vi "add channel to active arrayv2.vi"(0 "line array in":u32[](array[numeric]), 1 "line to add":u32) -> (2 "line array out":u32[](array[numeric]), 3 "addition":bool, 4 "index":i32)   [LabVIEW 2015]
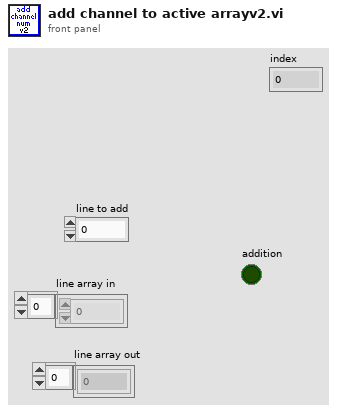
[diagram p1: front panel]
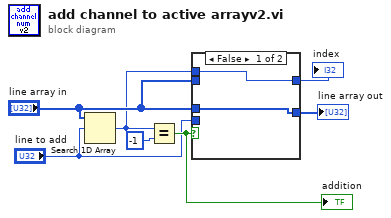
[diagram p0: block diagram]
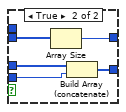
[diagram p2: hidden frame]
diagram:
  n1 = Search 1D Array(1D array="line array in", element="line to add") -> (index of element=w1:i32)  [unwired: 1 in]
  n2 = Equal?(x=w1, y=-1) -> (x = y?=w5:bool)
  "addition" <- w5
  n3 = case shown="False" w5 {
    tunnel: "line to add" -> [_ w13]
    tunnel: "line array in" -> [w9 w14]
    tunnel: [w9 w12] -> w7
    tunnel: "line array in" -> [_ w11]
    tunnel: [w8 w10] -> w2
    tunnel: w1 -> [w8 _]
    frame False {
    }
    frame True {
      n4 = Array Size(array=w11) -> (size(s)=w10:i32)
      n5 = Build Array (concatenate)(w14, w13) -> (w12:u32[])
    }
  }
  "line array out" <- w7
  "index" <- w2
